vi "Load e-series.vi"(8 "error in (no error)":errorcluster, 11 "INI File":string="e-series files names.ini") -> (0 "error out":errorcluster, 3 "E Series":T1)   [LabVIEW 2018, in "E Series Reader.lvlib"]
uses:
  E Series Reader.lvlib
  Data--control.ctl
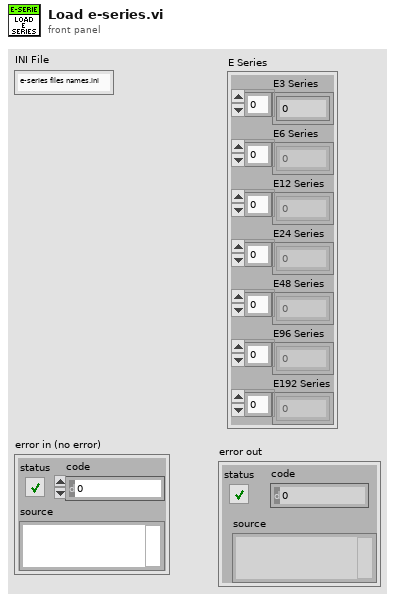
[diagram p1: front panel]
types:
  T1 = typedef "E Series Reader.lvlib/Data--control.ctl" = cluster{"E3 Series":u16[], "E6 Series ":u16[], "E12 Series":u16[], "E24 Series":u16[], "E48 Series":u16[], "E96 Series":u16[], "E192 Series":u16[]}
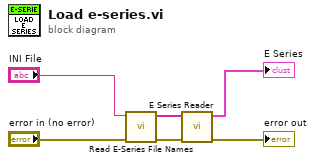
[diagram p0: block diagram]
diagram:
  n1 = call "Read E-Series File Names.vi"("error in (no error)"="error in (no error)", "INI File"="INI File") -> ("error out"=w5:errorcluster, "E-Series File Names"=w6:string[])  [unwired: 8 in]
  n2 = call "E Series Reader.vi"("error in"=w5, "File name"=w6) -> ("error out"=→"error out":errorcluster, "E Series"=→"E Series":T1)  [unwired: 8 in]
